vi "Enum Dev.vi"(0 "enumfilter":i32, 11 "error in (no error)":errorcluster) -> (2 "DeviceVersion":i32[](array[numeric]), 3 "isBusy":i32[](array[numeric]), 4 "pnDevice":i32, 6 "DevName":string[](array[string]), 8 "SN":string[](array[string]), 10 "UserName":string[](array[string]), 14 "DeviceID":i32[](array[numeric]), 15 "error out":errorcluster)   [LabVIEW 2014, in "AnalogDiscSDKLv.lvlib"]
doc: "extern \"C\" __declspec(dllexport) int Enum_DevLv(ENUMFILTER enumfilter, \n int * pnDevice, char DevName[MAX_DEVICE_NUMBER][DEVICE_INFO_STRING_LENGTH], char SN[MAX_DEVICE_NUMBER][DEVICE_INFO_STRING_LENGTH], char UserName[MAX_DEVICE_NUMBER][DEVICE_INFO_STRING_LENGTH], int isBusy[MAX_DEVICE_NUMBER], DEVID DeviceID[MAX_DEVICE_NUMBER], DEVVER DeviceVersion[MAX_DEVICE_NUMBER] );"
uses:
  <instrlib>/AnalogDiscSDKLv/AnalogDiscSDKLv.lvlib
  <instrlib>/AnalogDiscSDKLv/AnalogDiscSDKLv.dll
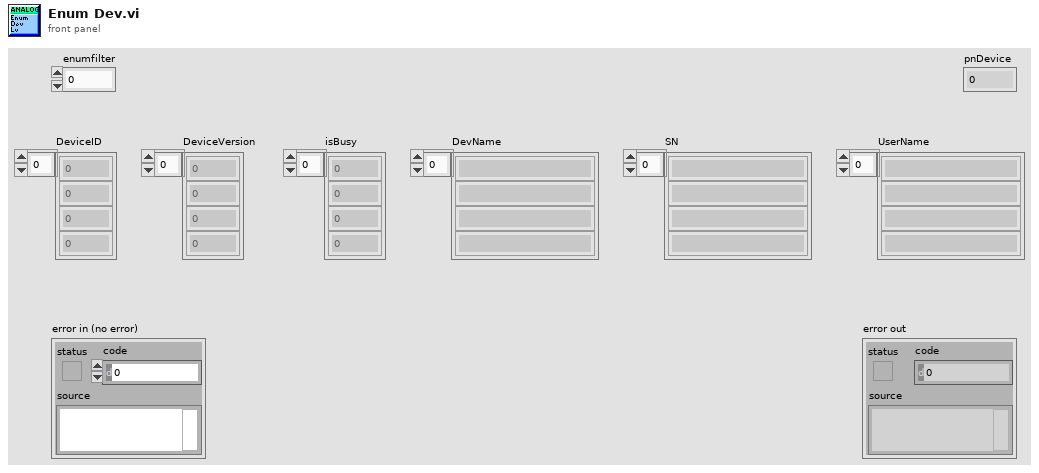
[diagram p1: front panel]
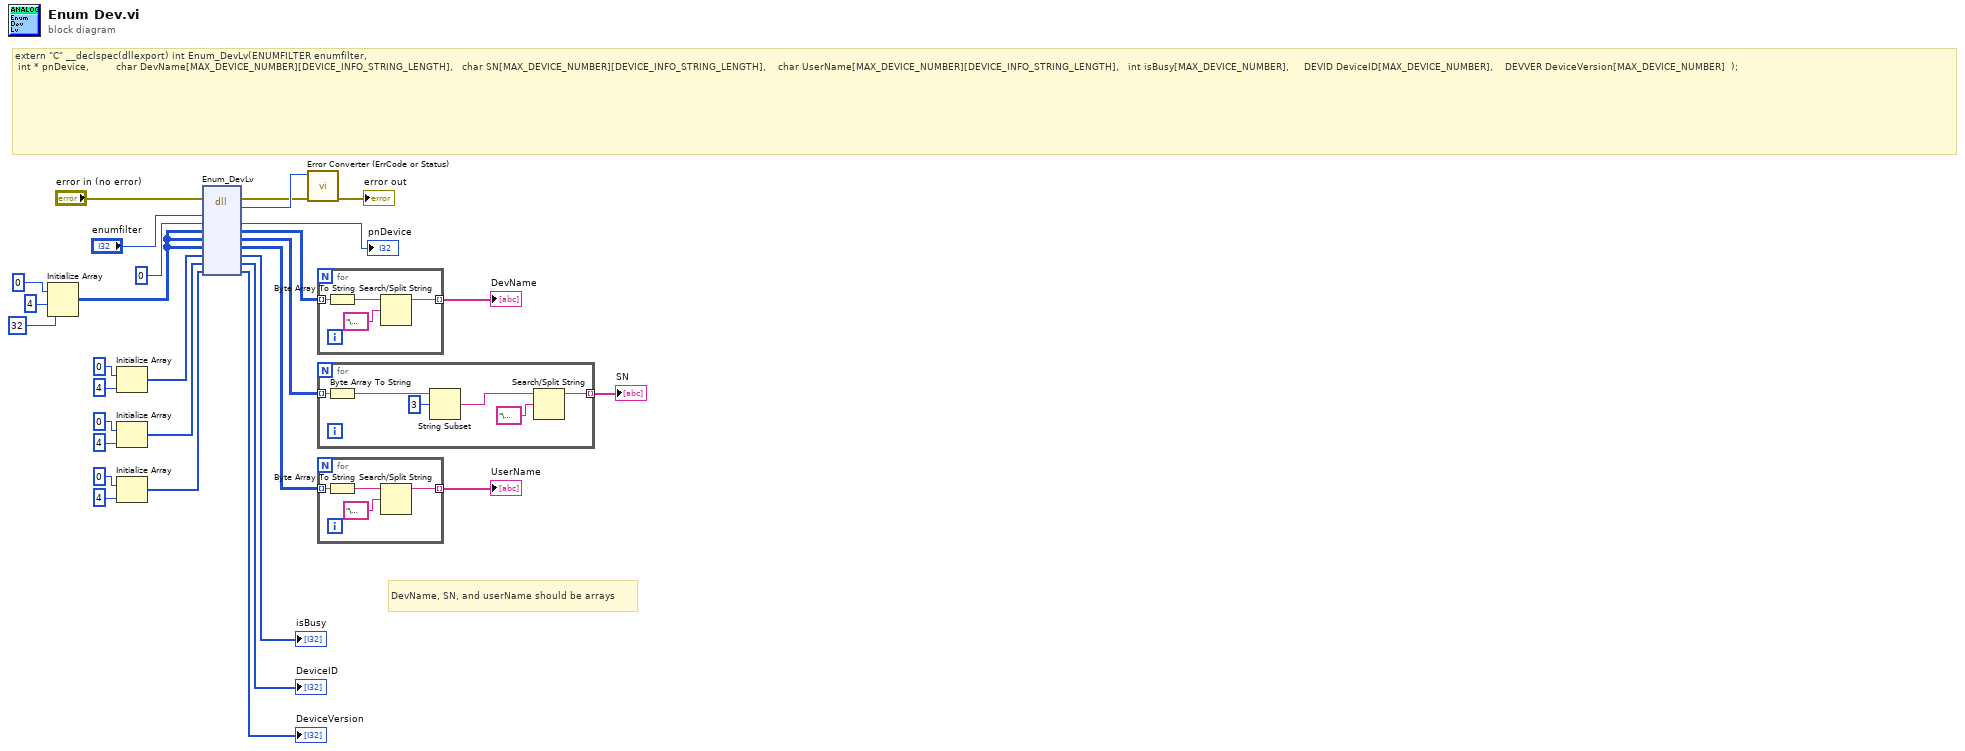
[diagram p0: block diagram]
diagram:
  # "DevName, SN, and userName should be arrays"
  # "extern \"C\" __declspec(dllexport) int Enum_DevLv(ENUMFILTER enumfilter, \n\tint * pnDevice,\t\t\t\t\t\t\t\t\tchar DevName[MAX_DEVICE_NUMBER][DEVICE_INFO_STRING_LENGTH],\t\t\tchar SN[MAX_DEVICE_NUMBER][DEVICE_INFO_STRING_LENGTH],\t\t\t\tchar UserName[MAX_DEVICE_NUMBER][DEVICE_INFO_STRING_LENGTH],\t\t\tint isBusy[MAX_DEVICE_NUMBER],\t\t\t\t\tDEVID DeviceID[MAX_DEVICE_NUMBER],\t\t\t\tDEVVER DeviceVersion[MAX_DEVICE_NUMBER]\t\t);"
  n1 = Initialize Array(u8 0 ("element"), 4 ("dimension size"), 32 ("dimension size")) -> (w7:u8[][])
  n2 = Initialize Array(0 ("element"), 4 ("dimension size")) -> (w23:i32[])
  n3 = Initialize Array(0 ("element"), 4 ("dimension size")) -> (w19:i32[])
  n4 = Initialize Array(0 ("element"), 4 ("dimension size")) -> (w15:i32[])
  n5 = dll-call lib="C:/Program Files (x86)/National Instruments/LabVIEW 2014/instr.lib/AnalogDiscSDKLv/AnalogDiscSDKLv.*" fn="Enum_DevLv"(error in="error in (no error)", "enumfilter"="enumfilter", "pnDevice"=0, "DevName"=w7, "SN"=w7, "UserName"=w7, "isBusy"=w23, "DeviceID"=w19, "DeviceVersion"=w15) -> (error out=w10:errorcluster, "return type"=w29:i32, "pnDevice"=→"pnDevice":i32, "DevName"=w6:u8[][], "SN"=w4:u8[][], "UserName"=w3:u8[][], "isBusy"=→"isBusy":i32[], "DeviceID"=→"DeviceID":i32[], "DeviceVersion"=→"DeviceVersion":i32[])  [unwired: 3 in, 1 out]
  n6 = call <instrlib>:"Error Converter (ErrCode or Status).vi"("error in (no error)"=w10, "error code"=w29) -> ("error out"=→"error out":errorcluster)  [unwired: 9 in]
  n7 = for {
    tunnel: [w30] -> w5 mode=indexing
    tunnel: w6 -> [w33] mode=indexing
    n8 = Byte Array To String(unsigned byte array=w33) -> (string=w32:string)
    n9 = Search/Split String(string=w32, search string/char (-)="\u0000") -> (substring before match=w30:string)  [unwired: 1 in, 2 out]
  }
  "DevName" <- w5
  n10 = for {
    tunnel: [w37] -> w1 mode=indexing
    tunnel: w4 -> [w39] mode=indexing
    n11 = Byte Array To String(unsigned byte array=w39) -> (string=w36:string)
    n12 = String Subset(string=w36, offset (0)=3) -> (substring=w35:string)  [unwired: 1 in]
    n13 = Search/Split String(string=w35, search string/char (-)="\u0000") -> (substring before match=w37:string)  [unwired: 1 in, 2 out]
  }
  "SN" <- w1
  n14 = for {
    tunnel: [w40] -> w2 mode=indexing
    tunnel: w3 -> [w43] mode=indexing
    n15 = Byte Array To String(unsigned byte array=w43) -> (string=w42:string)
    n16 = Search/Split String(string=w42, search string/char (-)="\u0000") -> (substring before match=w40:string)  [unwired: 1 in, 2 out]
  }
  "UserName" <- w2
